vi "HeaderAction.vi"(0 "InstrClass":refnum<class "LSCI332.lvclass"> caption="DNL_LabVIEW Object in", 11 "error in (no error)":errorcluster caption="entrée d'erreur (pas d'erreur)") -> (4 "InstrClassOut":refnum<class "LSCI332.lvclass"> caption="DNL_LabVIEW Object out", 6 "DataNames":string[](array[string]), 8 "Instr Name":string, 10 "HeaderString":string, 13 "ArrDisplayNames":string[](array[string]), 14 "DisplayNames":string[](array[string]), 15 "error out":errorcluster caption="sortie d'erreur")   [LabVIEW 2019, in "LSCI332.lvclass"]
uses:
  LSCI332.lvclass
  C:/Programmes LabView/LabScanV1A/DevicesClass/BaseDevice/BaseDevice.lvclass
  LSCI332.lvclass/LSCI332.ctl
  <userlib>/LSCI 332 V2/GetAllPAr States.ctl
  BaseDevice/BaseDevice.lvclass
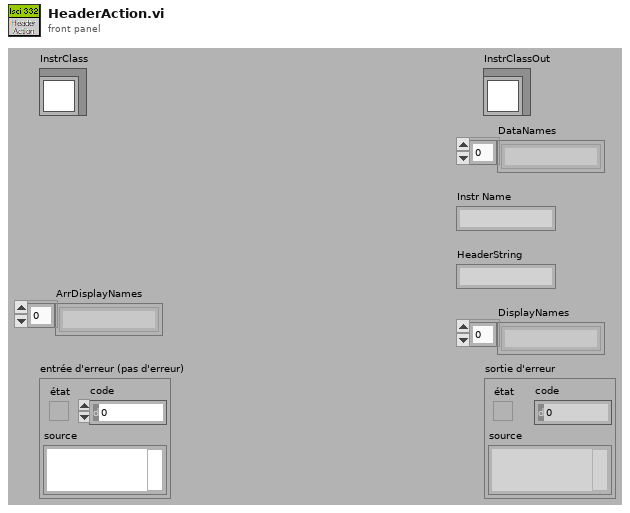
[diagram p1: front panel]
types:
  T1 = typedef "GetAllPAr States.ctl" = enum16{"Input A Par", "Input B Par", "Heater Params", "Loop 1 Par", "Loop 2 Par", "All"}
  T2 = typedef "LSCI332.lvclass/LSCI332_Func.ctl" = enum16{"Read_InputA (K,S)", "Read_InputA&Heater (K,S,%,W)", "Read_InputB (K,S)", "Read_InputB&Heater (K,S,%,W)", "Read_Heater (%,W)", "Read_InputA&B(K,S,K,S)", "Read_InputA&B&Heater (K,S,K,S,%,W)", "Scan_Loop1(K,S)", "Scan_Loop2(K,S)"}
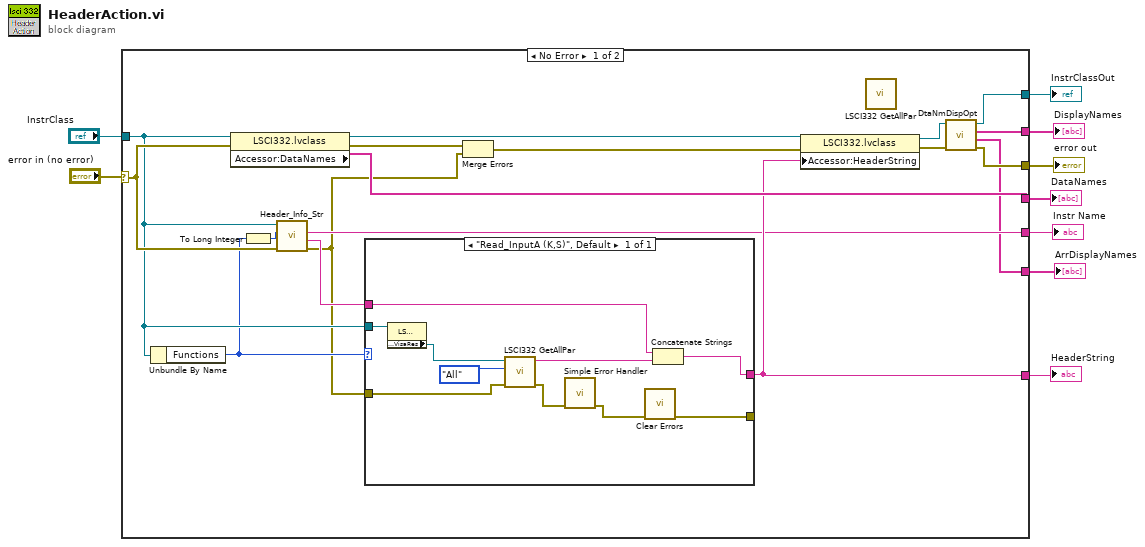
[diagram p0: block diagram]
diagram:
  n1 = case shown="No Error" "error in (no error)" {
    selector: "error in (no error)" -> [w16 w38]
    tunnel: [w24 _] -> w8
    tunnel: [w27 _] -> w7
    tunnel: "InstrClass" -> [w14 w39]
    tunnel: [w22 w38] -> w5
    tunnel: [w21 w39] -> w3
    tunnel: [w18 _] -> w4
    tunnel: [w19 _] -> w2
    tunnel: [w11 _] -> w1
    frame No Error {
      n2 = Unbundle By Name(w14) -> ("Functions"=w13:T2)
      n3 = property class="LSCI332.lvclass"(reference=w14, error in=w16) -> (reference out=w26:refnum<class "LSCI332.lvclass">, error out=w25:errorcluster, "Accessor:DataNames"=w27:string[])
      n4 = To Long Integer(number=w13) -> (32bit integer=w12:i32)
      n5 = call-dynamic "Header_Info_Str.vi"("error in (no error)"=w16, "Functions"=w12, "DefaultDev in"=w14) -> ("error out"=w10:errorcluster, "HdrInfoStr"=w17:string, "InstrumentName"=w18:string)  [unwired: 5 in, 1 out]
      n6 = case shown="\"Read_InputA (K,S)\", Default" w13 {
        tunnel: [w31] -> w24
        tunnel: w17 -> [w34]
        tunnel: w14 -> [w37]
        tunnel: w10 -> [w36]
        tunnel: [w28] -> _
        frame "Read_InputA (K,S)", Default {
          n7 = property class="LSCI332.lvclass"(reference=w37) -> ("Accessor:VisaRes"=w32:refnum<visa-resource-name>)  [unwired: 1 in, 2 out]
          n8 = call <userlib>:"LSCI332 GetAllPar.vi"("error in"=w36, "Parameters"=GetAllPAr_States."All", "VISA Rsrc"=w32) -> ("error out"=w30:errorcluster, "Parameter String"=w35:string)  [unwired: 5 in]
          n9 = call <vilib>:"Simple Error Handler.vi"("error in (no error)"=w30) -> ("error out"=w29:errorcluster)  [unwired: 4 in, 4 out]
          n10 = call <vilib>:"Clear Errors.vi"("error in (no error)"=w29) -> ("error out"=w28:errorcluster)  [unwired: 5 in, 1 out]
          n11 = Concatenate Strings(w34, w35) -> (w31:string)
        }
      }
      n12 = Merge Errors(w25, w10) -> (w15:errorcluster)
      n13 = property class="LSCI332.lvclass"(reference=w26, error in=w15, "Accessor:HeaderString"=w24) -> (reference out=w20:refnum<class "LSCI332.lvclass">, error out=w23:errorcluster)
      n14 = call <userlib>:"LSCI332 GetAllPar.vi"() -> ()  [unwired: 8 in, 2 out]
      n15 = call "DtaNmDispOpt.vi"("error in (no error)"=w23, "BaseDevice en entrée"=w20) -> ("error out"=w22:errorcluster, "ArrDisplayNames"=w11:string[], "DisplayNames"=w19:string[], "BaseDevice en sortie"=w21:refnum<class "LSCI332.lvclass">)  [unwired: 6 in]
    }
    frame Error {
    }
  }
  "error out" <- w5
  "InstrClassOut" <- w3
  "DataNames" <- w7
  "HeaderString" <- w8
  "Instr Name" <- w4
  "DisplayNames" <- w2
  "ArrDisplayNames" <- w1
